vi "Send Text Using SMTP API 2013 NIVerified.vi"(4 "Body":string, 5 "Carrier":T1(ring), 6 "Subject":string, 7 "phone number":string, 10 "Password":string, 11 "Email":string) -> ()   [LabVIEW 2017]
uses:
  <vilib>/smtpClient/Set Message Text.vi
  <vilib>/smtpClient/LabVIEWSMTPClient.lvlib
panel:
  in  "TLS":bool=TRUE
  in  "Outgoing Mail Server (SMTP)":string="smtp.gmail.com"
  # "Overview\nThis example will allows you to use an SMTP server to send a SMS message to a cell phone.\nDescription\nWith the SMTP API you can send an email to your phone as a text message.  There are a lot of different servers you\n can use the default in this example is using GMAIL through the smtp.gmail.com server.  Most SMTP servers should \nwork, but the server and cell phone needs to be compatible to send and receive SMS messages.\nSteps to Implement or Execute Code\nOpen Send Text using SMTP API.vi\nFill in the SMTP server in the Outgoing Mail Server (SMTP), gmail is the default server\nFill out your email & Password\nSelect your Carrier and Type your Phone Number\nType the text you would like to send in the Body Control"
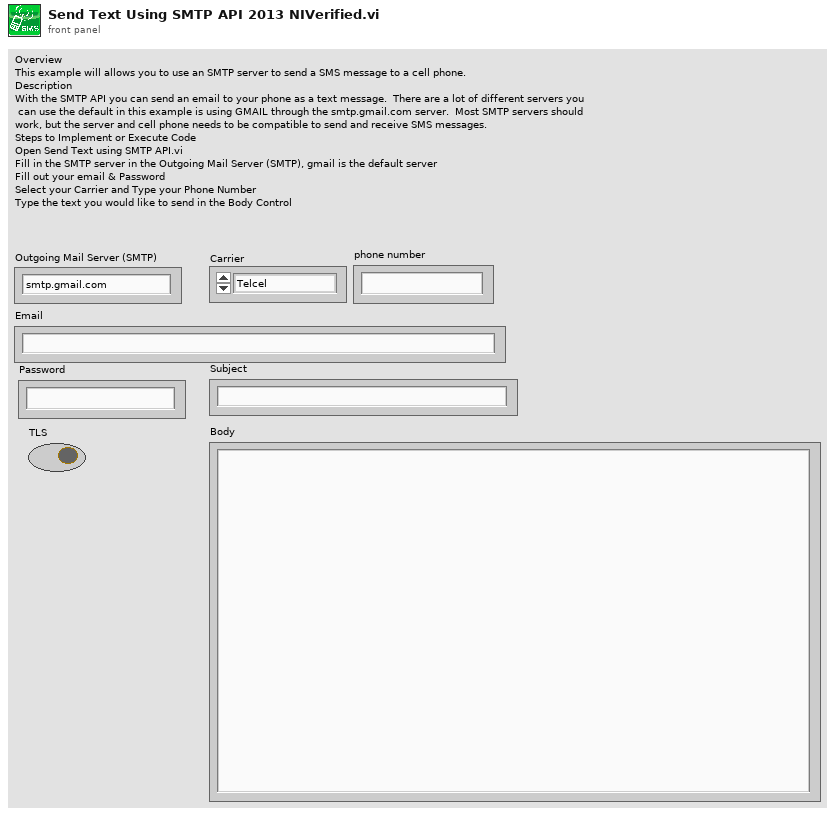
[diagram p1: front panel]
types:
  T1 = enum16{"Telcel", "T-Mobile", "AT&T", "Verizon", "Sprint"}
  T2 = typedef "LabVIEWSMTPClient.lvlib/SmtpClientHandle.ctl" = refnum<k1>
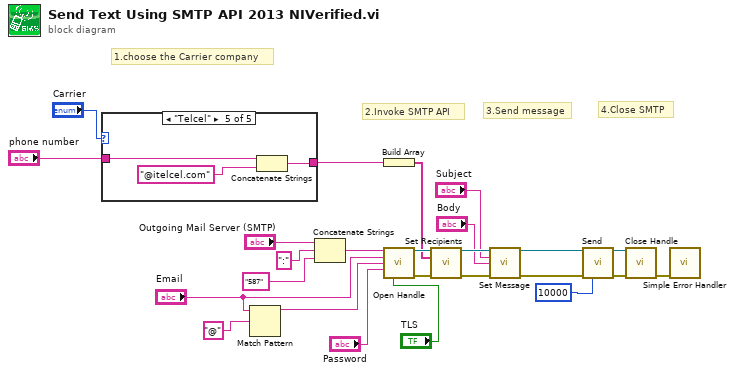
[diagram p0: block diagram]
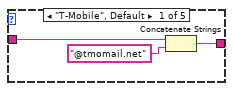
[diagram p2: hidden frame]
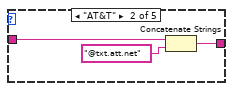
[diagram p3: hidden frame]
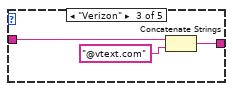
[diagram p4: hidden frame]
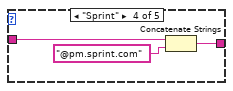
[diagram p5: hidden frame]
diagram:
  # "4.Close SMTP"
  # "3.Send message"
  # "2.Invoke SMTP API"
  # "1.choose the Carrier company"
  n1 = case shown="\"Telcel\"" "Carrier" {
    tunnel: "phone number" -> [w28 w30 w33 w36 w38]
    tunnel: [w26 w31 w34 w37 w40] -> w12
    frame "T-Mobile", Default {
      n2 = Concatenate Strings(w28, "@tmomail.net" ("string")) -> (w26:string)
    }
    frame "AT&T" {
      n3 = Concatenate Strings(w30, "@txt.att.net" ("string")) -> (w31:string)
    }
    frame "Verizon" {
      n4 = Concatenate Strings(w33, "@vtext.com" ("string")) -> (w34:string)
    }
    frame "Sprint" {
      n5 = Concatenate Strings(w36, "@pm.sprint.com") -> (w37:string)
    }
    frame "Telcel" {
      n6 = Concatenate Strings(w38, "@itelcel.com" ("string")) -> (w40:string)
    }
  }
  n7 = Match Pattern(string="Email", regular expression="@") -> (before substring=w1:string)  [unwired: 1 in, 3 out]
  n8 = Concatenate Strings("Outgoing Mail Server (SMTP)", ":" ("string"), "587" ("Port")) -> (w7:string)
  n9 = Build Array(w12) -> (w11:string[])
  n10 = call <vilib>:"Open Handle.vi"("server address"=w7, "from"="Email", "username"=w1, "password"="Password", "use TLS (false)"="TLS") -> ("handle out"=w23:T2, "error out"=w21:errorcluster)  [unwired: 9 in]
  n11 = call <vilib>:"Set Recipients.vi"("handle in"=w23, "to"=w11, "error in (no error)"=w21) -> ("handle out"=w20:T2, "error out"=w19:errorcluster)  [unwired: 11 in]
  n12 = call-poly <vilib>:"Set Message.vi"("handle in"=w20, "subject"="Subject", "plain text message"="Body", "error in (no error)"=w19) -> ("handle out"=w16:T2, "error out"=w15:errorcluster)  [unwired: 10 in]
  n13 = call <vilib>:"Send.vi"("handle in"=w16, "error in (no error)"=w15, "timeout in ms (10000)"=10000) -> ("handle out"=w14:T2, "error out"=w13:errorcluster)  [unwired: 10 in, 1 out]
  n14 = call <vilib>:"Close Handle.vi"("handle in"=w14, "error in (no error)"=w13) -> ("error out"=w4:errorcluster)  [unwired: 12 in, 1 out]
  n15 = call <vilib>:"Simple Error Handler.vi"("error in (no error)"=w4) -> ()  [unwired: 4 in, 5 out]
